vi "Sample_Event_Handler.vi"() -> ()   [LabVIEW 2022 SP3]
uses:
  <vilib>/numeric/Random Number (Range) DBL.vi
panel:
  in  "Continuous Generation":bool
  out "Current Event":string
  in  "Stop":bool
  in  "Generate":bool
  in  "Timeout":i32=50
  out "Waveform Chart":dbl[](graph)
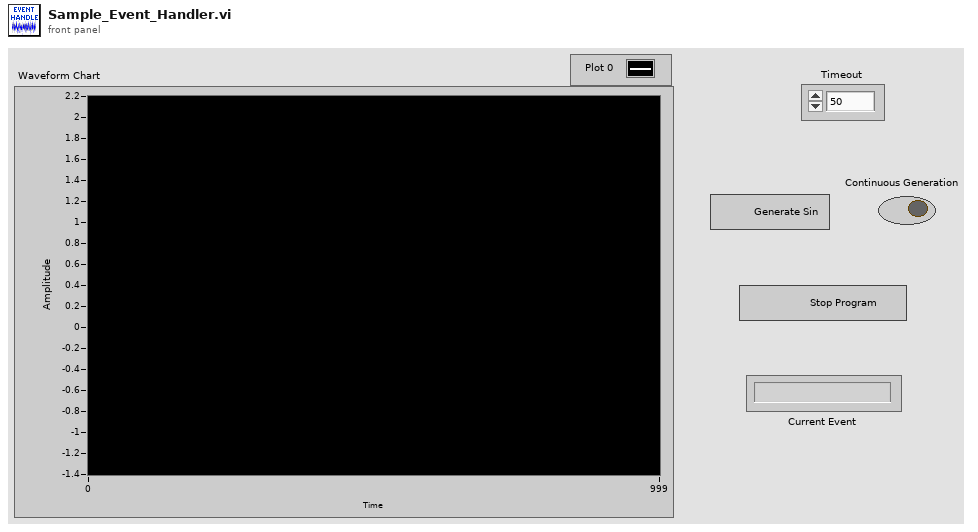
[diagram p1: front panel]
types:
  T1 = enum8{"Enabled", "Disabled", "Disabled and Grayed Out"}
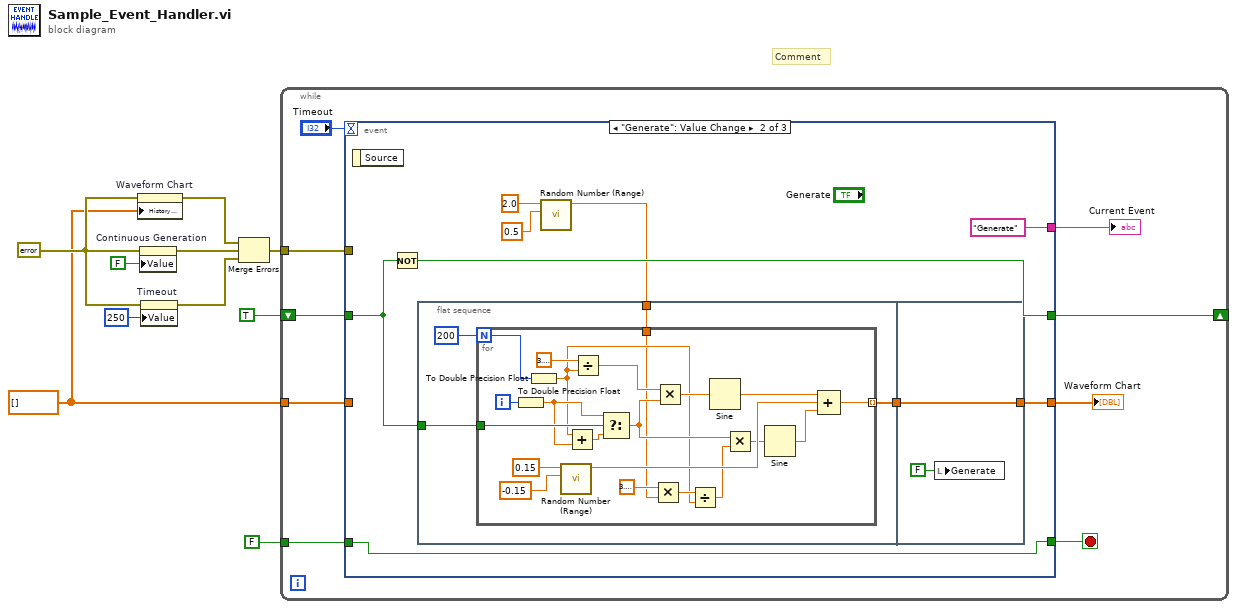
[diagram p0: block diagram]
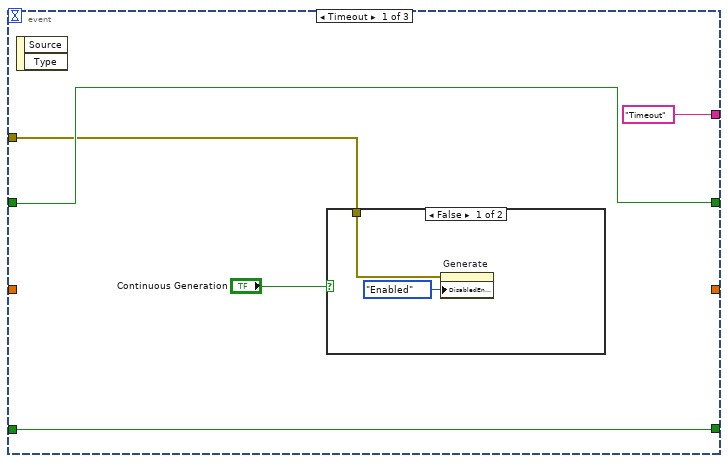
[diagram p2: hidden frame]
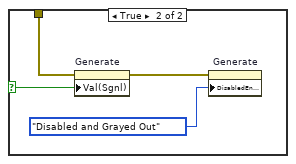
[diagram p3: hidden frame]
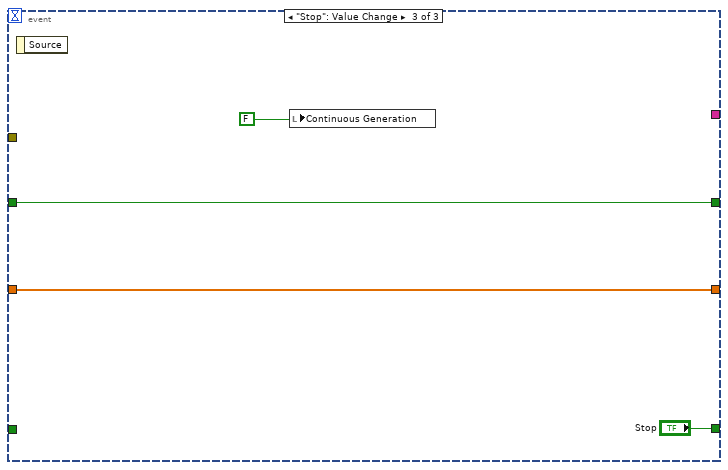
[diagram p4: hidden frame]
diagram:
  w3 = errorcluster {"status"=FALSE, "code"=0, "source"=""} ("error in (no error)")
  w2 = dbl[] []
  # "Comment"
  n1 = property on="Waveform Chart" class="WFChart (strict)"(error in=w3, "History Data"=w2) -> (error out=w1:errorcluster)  [unwired: 1 in, 1 out]
  n2 = property on="Continuous Generation" class="Bool (strict)"(error in=w3, "Value"=FALSE ("Continuous Generation")) -> (error out=w7:errorcluster)  [unwired: 1 in, 1 out]
  n3 = property on="Timeout" class="DigNum (strict)"(error in=w3, "Value"=250 ("Timeout")) -> (error out=w6:errorcluster)  [unwired: 1 in, 1 out]
  n4 = Merge Errors(w1, w7, w6) -> (w8:errorcluster)
  n5 = while {
    tunnel: FALSE ("Generate") -> [w17]
    tunnel: w2 -> [w16]
    shift-right: [w12] -> _
    shift-left: TRUE -> [w13]
    tunnel: w8 -> [w11]
    stop <- w18 stop-if-true
    n6 = event shown="[1] \"Generate\": Value Change" {
      selector: _ -> [_ _ _]
      dyn-events: _ -> [_ _ _]
      timeout: "Timeout" -> [_ _ _]
      tunnel: [w24 w36 "Stop"] -> w18
      tunnel: w17 -> [w24 w36 _]
      tunnel: [_ w39 w69] -> w15
      tunnel: w16 -> [_ _ w69]
      tunnel: ["Timeout" ("State") "Generate" ("State") _] -> w14
      tunnel: w13 -> [w22 w35 w68]
      tunnel: [w22 w37 w68] -> w12
      tunnel: w11 -> [w20 _ _]
      event Timeout {
        n7 = event-data() -> ()  [unwired: 1 in, 2 out]
        n8 = case shown="False" "Continuous Generation" {
          selector: "Continuous Generation" -> [_ w29]
          tunnel: w20 -> [w26 w30]
          frame False {
            n9 = property on="Generate" class="Bool (strict)"(error in=w26, "DisabledEnum"=T1."Enabled" ("Disabled")) -> ()  [unwired: 1 in, 2 out]
          }
          frame True {
            n10 = property on="Generate" class="Bool (strict)"(error in=w30, "Val(Sgnl)"=w29) -> (error out=w28:errorcluster)  [unwired: 1 in, 1 out]
            n11 = property on="Generate" class="Bool (strict)"(error in=w28, "DisabledEnum"=T1."Disabled and Grayed Out" ("Disabled")) -> ()  [unwired: 1 in, 2 out]
          }
        }
      }
      event "Generate": Value Change {
        n12 = event-data() -> ()  [unwired: 1 in, 1 out]
        n13 = Not(x=w35) -> (.not. x?=w37:bool)
        n14 = flat-sequence {
          tunnel: w35 -> [w41]
          tunnel: [w42] -> w34
          tunnel: w31 -> [w40]
          tunnel: [w66] -> w39
          tunnel: w34 -> [w66]
          frame #0 {
            n15 = for {
              N: 200 -> [w64]
              tunnel: [w49] -> w42 mode=indexing
              tunnel: w41 -> [w58]
              tunnel: w40 -> [w44]
              i -> [w62]
              n16 = To Double Precision Float(number=w62) -> (double precision float=w57:dbl)
              n17 = To Double Precision Float(number=w64) -> (double precision float=w46:dbl)
              n18 = call-poly <vilib>:"Random Number (Range).vi"("lower bound (0)"=-0.15 ("upper bound (100)"), "upper bound (100)"=0.15) -> ("number"=w53:dbl)  [unwired: 9 in]
              n19 = Add(x=w46, y=w57) -> (x+y=w56:dbl)
              n20 = Divide(x=3.141592653589793, y=w46) -> (x/y=w63:dbl)
              n21 = Select(t=w57, s=w58, f=w56) -> (s? t:f=w52:dbl)
              n22 = Multiply(x=3.141592653589793, y=w44) -> (x*y=w47:dbl)
              n23 = Multiply(x=w63, y=w52) -> (x*y=w61:dbl)
              n24 = Divide(x=w47, y=w46) -> (x/y=w45:dbl)
              n25 = Sine(x=w61) -> (sin(x)=w54:dbl)
              n26 = Multiply(x=w52, y=w45) -> (x*y=w51:dbl)
              n27 = Sine(x=w51) -> (sin(x)=w50:dbl)
              n28 = Compound Arithmetic op=ADD(w54, w53, w50) -> (w49:dbl)
            }
          }
          frame #1 {
            n29 = local write "Generate"(FALSE ("Generate")) -> ()
          }
        }
        n30 = call-poly <vilib>:"Random Number (Range).vi"("lower bound (0)"=0.5, "upper bound (100)"=2.0) -> ("number"=w31:dbl)  [unwired: 9 in]
      }
      event "Stop": Value Change {
        n31 = event-data() -> ()  [unwired: 1 in, 1 out]
        n32 = local write "Continuous Generation"(FALSE ("Timeout Generation")) -> ()
      }
    }
    "Waveform Chart" <- w15
    "Current Event" <- w14
  }
